vi "motors_enable_disable.vi"(8 "Error In":errorcluster, 10 "Status":enum16{"Disable", "Enable"}(ring), 11 "VISA resource name":refnum<visa-resource-name>) -> (0 "Error Out":errorcluster, 3 "VISA resource name out":refnum<visa-resource-name>)   [LabVIEW 2019]
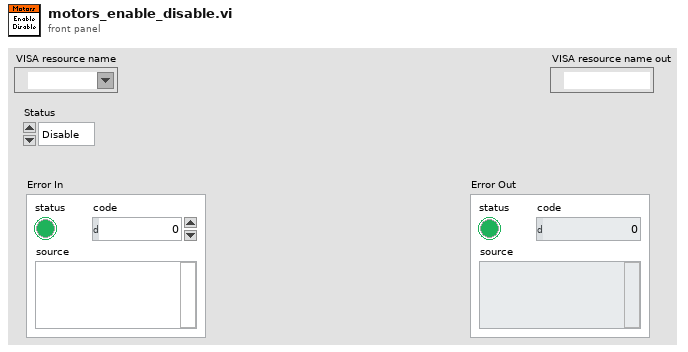
[diagram p1: front panel]
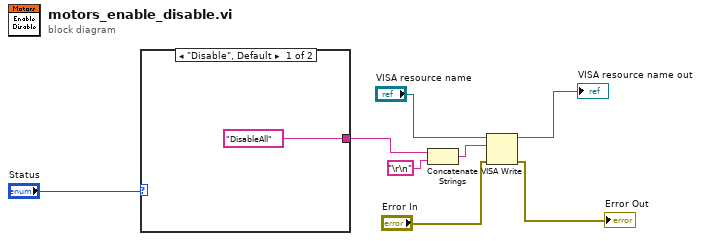
[diagram p0: block diagram]
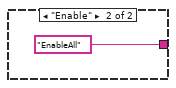
[diagram p2: hidden frame]
diagram:
  n1 = case shown="\"Disable\", Default" "Status" {
    tunnel: ["DisableAll" "EnableAll"] -> w5
    frame "Disable", Default {
    }
    frame "Enable" {
    }
  }
  n2 = Concatenate Strings(w5, "\r\n") -> (w6:string)
  n3 = VISA Write(VISA resource name="VISA resource name", write buffer=w6, error in (no error)="Error In") -> (VISA resource name out=→"VISA resource name out":refnum<visa-resource-name>, error out=→"Error Out":errorcluster)  [unwired: 1 out]
